vi "Is dependency.vi"(8 "error in (no error)":errorcluster, 11 "VI Reference":refnum<vi>) -> (0 "error out":errorcluster, 3 "Is project dependency":bool)   [LabVIEW 2021]
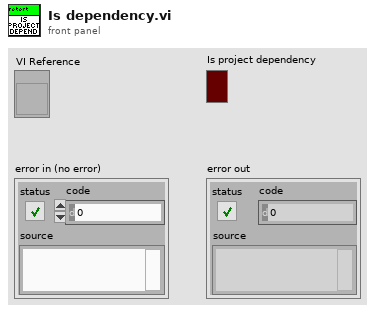
[diagram p1: front panel]
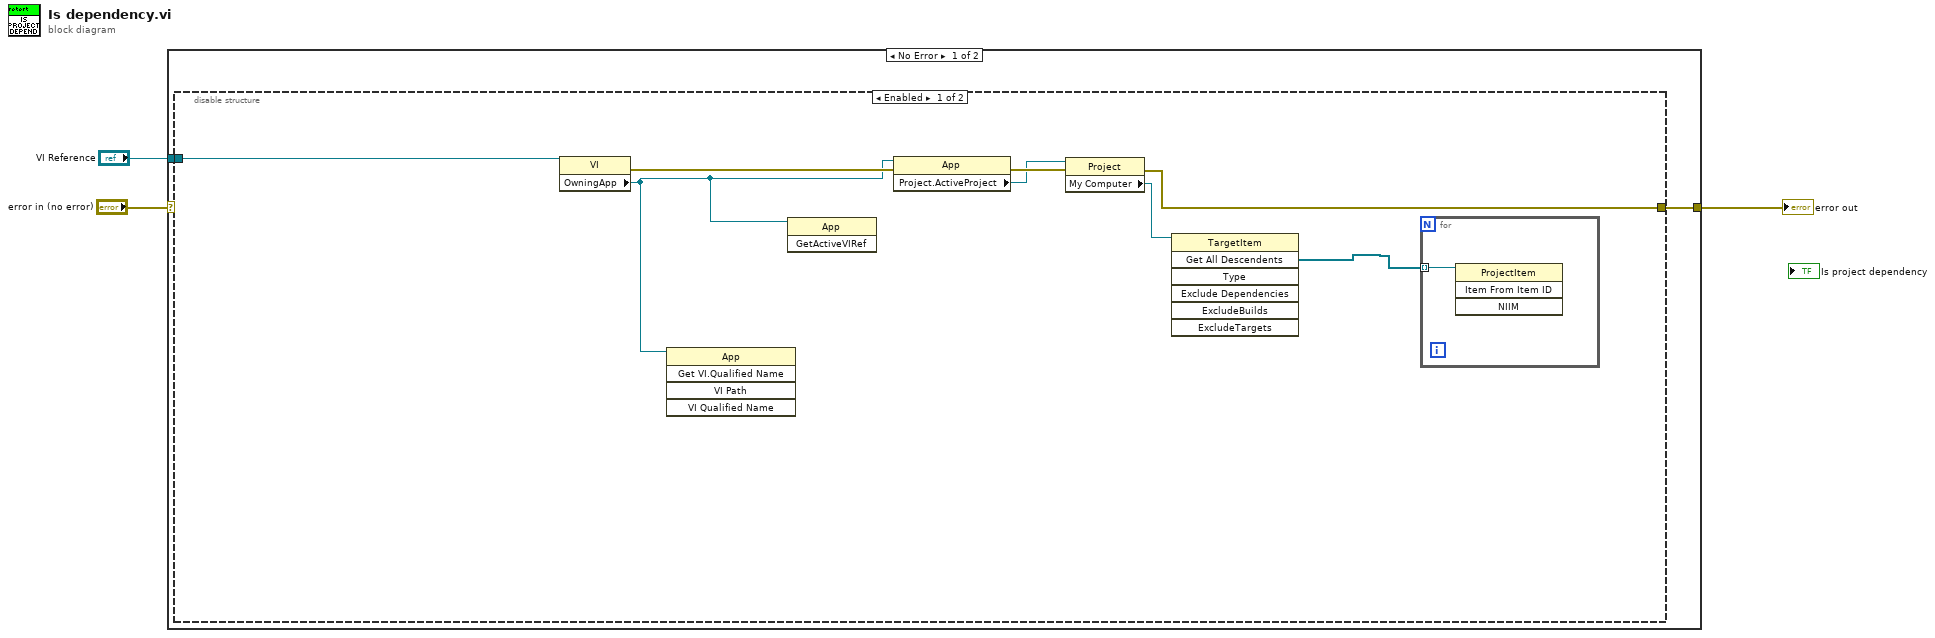
[diagram p0: block diagram]
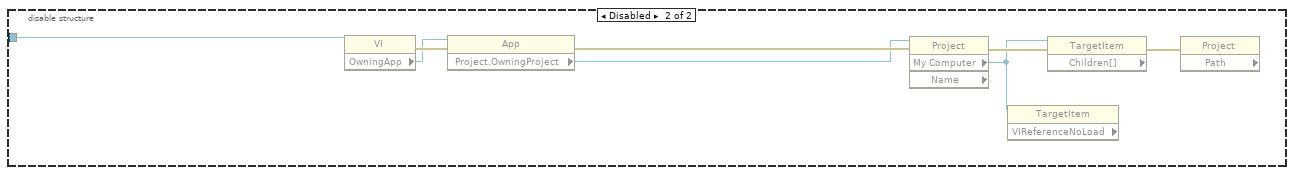
[diagram p2: hidden frame]
diagram:
  n1 = case shown="No Error" "error in (no error)" {
    selector: "error in (no error)" -> [_ w24]
    tunnel: "VI Reference" -> [w5 _]
    tunnel: [w4 w24] -> w1
    frame No Error {
      n2 = disable-structure shown="Enabled" {
        disable-tunnel: w5 -> [w11 w21]
        disable-tunnel: [w13 _] -> w4
        frame Enabled {
          n3 = property class="VI"(reference=w11) -> (error out=w12:errorcluster, "OwningApp"=w10:refnum<vi>)  [unwired: 1 in, 1 out]
          n4 = invoke on="Invoke Node" class="App" method="Get VI.Qualified Name"(reference=w10) -> ()  [unwired: 4 in, 5 out]
          n5 = invoke on="Invoke Node" class="App" method="GetActiveVIRef"(reference=w10) -> ()  [unwired: 2 in, 3 out]
          n6 = property class="App"(reference=w10, error in=w12) -> (error out=w14:errorcluster, "Project.ActiveProject"=w8:refnum<vi>)  [unwired: 1 out]
          n7 = property class="Project"(reference=w8, error in=w14) -> (reference out=w9:refnum<vi>, error out=w13:errorcluster, "My Computer"=w7:refnum<vi>)
          n8 = invoke on="Invoke Node" class="TargetItem" method="Get All Descendents"(reference=w7) -> ("All Descendents"=w6:refnum<vi>[])  [unwired: 6 in, 6 out]
          n9 = for {
            tunnel: w6 -> [w15] mode=indexing
            n10 = invoke on="Invoke Node" class="ProjectItem" method="Item From Item ID"(reference=w15) -> ()  [unwired: 3 in, 4 out]
          }
        }
        frame Disabled {
          n11 = property class="VI"(reference=w21) -> (error out=w23:errorcluster, "OwningApp"=w20:refnum<vi>)  [unwired: 1 in, 1 out]
          n12 = property class="App"(reference=w20, error in=w23) -> (error out=w22:errorcluster, "Project.OwningProject"=w17:refnum<vi>)  [unwired: 1 out]
          n13 = property class="Project" props=["My Computer", "Name"](reference=w17, error in=w22) -> (error out=w19:errorcluster, "My Computer"=w16:refnum<vi>)  [unwired: 2 out]
          n14 = property class="TargetItem" props=["VIReferenceNoLoad"](reference=w16) -> ()  [unwired: 1 in, 3 out]
          n15 = property class="TargetItem" props=["Children[]"](reference=w16, error in=w19) -> (error out=w18:errorcluster)  [unwired: 2 out]
          n16 = property class="Project" props=["Path"](error in=w18) -> ()  [unwired: 1 in, 3 out]
        }
      }
    }
    frame Error {
    }
  }
  "error out" <- w1
